vi "TrayitemCaculate.vi"(8 "error in":errorcluster, 11 "TrayType":T1) -> (0 "error out":errorcluster, 3 "item":i32)   [LabVIEW 2015]
uses:
  Tray/Tray_TrayName.ctl
  global/Tray_ArrAndData.vi
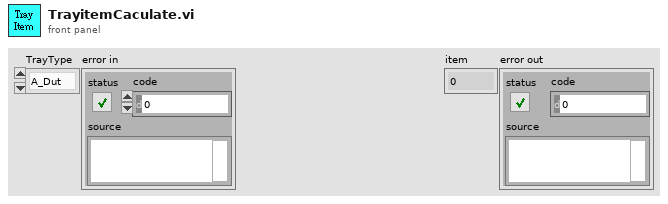
[diagram p1: front panel]
types:
  T1 = typedef "Tray_TrayName.ctl" = enum16{"A_Dut", "B_Pass", "C_NGR", "D_NGL"}
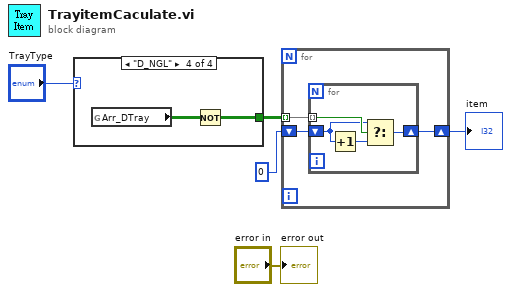
[diagram p0: block diagram]
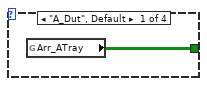
[diagram p2: hidden frame]
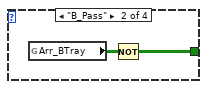
[diagram p3: hidden frame]
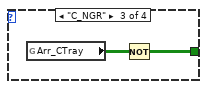
[diagram p4: hidden frame]
diagram:
  n1 = case shown="\"D_NGL\"" "TrayType" {
    tunnel: [w6 w7 w9 w11] -> w5
    frame "A_Dut", Default {
      n2 = global read "Tray_ArrAndData.vi" "Arr_ATray"() -> (w6:bool[][])
    }
    frame "B_Pass" {
      n3 = global read "Tray_ArrAndData.vi" "Arr_BTray"() -> (w8:bool[][])
      n4 = Not(x=w8) -> (.not. x?=w7:bool[][])
    }
    frame "C_NGR" {
      n5 = global read "Tray_ArrAndData.vi" "Arr_CTray"() -> (w10:bool[][])
      n6 = Not(x=w10) -> (.not. x?=w9:bool[][])
    }
    frame "D_NGL" {
      n7 = global read "Tray_ArrAndData.vi" "Arr_DTray"() -> (w12:bool[][])
      n8 = Not(x=w12) -> (.not. x?=w11:bool[][])
    }
  }
  n9 = for {
    tunnel: w5 -> [w15] mode=indexing
    shift-right: [w14] -> w3
    shift-left: 0 -> [w13]
    n10 = for {
      tunnel: w15 -> [w19] mode=indexing
      shift-right: [w18] -> w14
      shift-left: w13 -> [w17]
      n11 = Increment(x=w17) -> (x+1=w16:i32)
      n12 = Select(t=w17, s=w19, f=w16) -> (s? t:f=w18:i32)
    }
  }
  "item" <- w3
  "error out" <- "error in"
